vi "MB_TCP_7024i.vi"(5 "Status Reference":T1, 6 "N":i32, 7 "Data Reference":T2, 9 "timeouts":T3={"conn_timeout"=1000, "reconn_timeout"=3000, "N attempt max"=3, "t_reset_TTL"=120000, "write_timeout"=10, "read_timeout"=500, "period"=100} {"t_reset_TTL" min=10 max=240000 step=1; "period" min=10 max=100000 step=1; "read_timeout" min=10 max=60000 step=1; "write_timeout" min=1 max=60000 step=1; "N attempt max" min=1 max=5 step=1; "reconn_timeout" min=10 max=240000 step=1; "conn_timeout" min=10 max=240000}, 10 "write enable":bool=TRUE, 11 "stop":bool) -> (0 "error out":errorcluster, 2 "errors":i32, 3 "Z3":u32)   [LabVIEW 2019, in "MB_TCP1.lvlib"]
uses:
  MB_TCP1.lvlib
  Timer Delay/Timers.lvlib
  NI_modbus_upd/NI_modbus_upd.lvlib
  NI_modbus_upd/MB Modbus Command.ctl
  ICPCON Registers/ICPCON Registers.lvlib
  ICPCON Status/ICPCON Status.lvlib
  Timer Delay/unix time 1ms.vi
  NI_modbus_upd/TCP/TCP.lvclass
  ICPCON Status/Ctl/ICPCON Status.ctl
  ICPCON Registers/Ctl/ICPCON Data.ctl
panel:
  out "stopped":bool
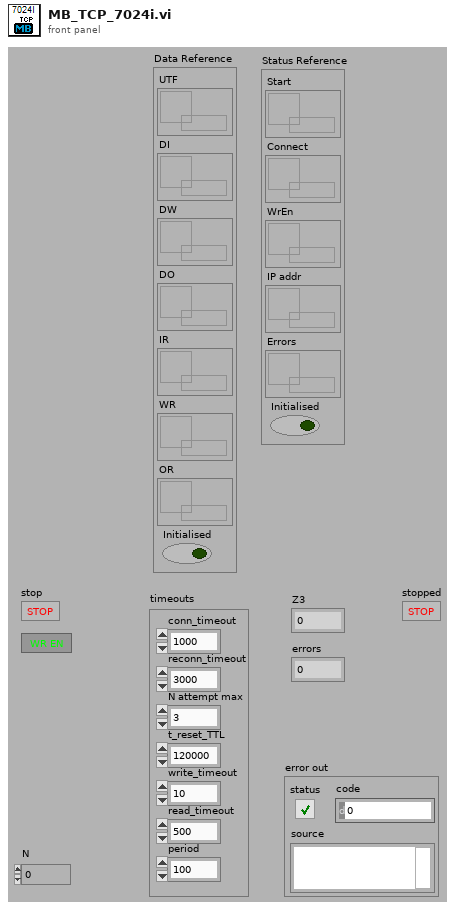
[diagram p1: front panel]
types:
  T1 = typedef "ICPCON Status.lvlib/ICPCON Status.ctl" = cluster{"Start":refnum<data-value>, "Connect":refnum<data-value>, "WrEn":refnum<data-value>, "IP addr":refnum<data-value>, "Errors":refnum<data-value>, "Initialised":bool}
  T2 = typedef "ICPCON Registers.lvlib/ICPCON Data.ctl" = cluster{"UTF":refnum<data-value>, "DI":refnum<data-value>, "DW":refnum<data-value>, "DO":refnum<data-value>, "IR":refnum<data-value>, "WR":refnum<data-value>, "OR":refnum<data-value>, "Initialised":bool}
  T3 = cluster{"conn_timeout":i32, "reconn_timeout":i32, "N attempt max":i32, "t_reset_TTL":i32, "write_timeout":i32, "read_timeout":i32, "period":i32}
  T4 = cluster{"Transaction ID":u16, "Protocol ID":u16, "Length":u16, "Unit ID":u8}
  T5 = typedef "NI_modbus_upd.lvlib/MB Modbus Command.ctl" = cluster{"Function Code":u8, "Starting Address":u16, "Quantity":u16, "Data":u16[], "Discrete":bool[]}
  T6 = cluster{"Remote IP Address":string, "Remote Port":u16}
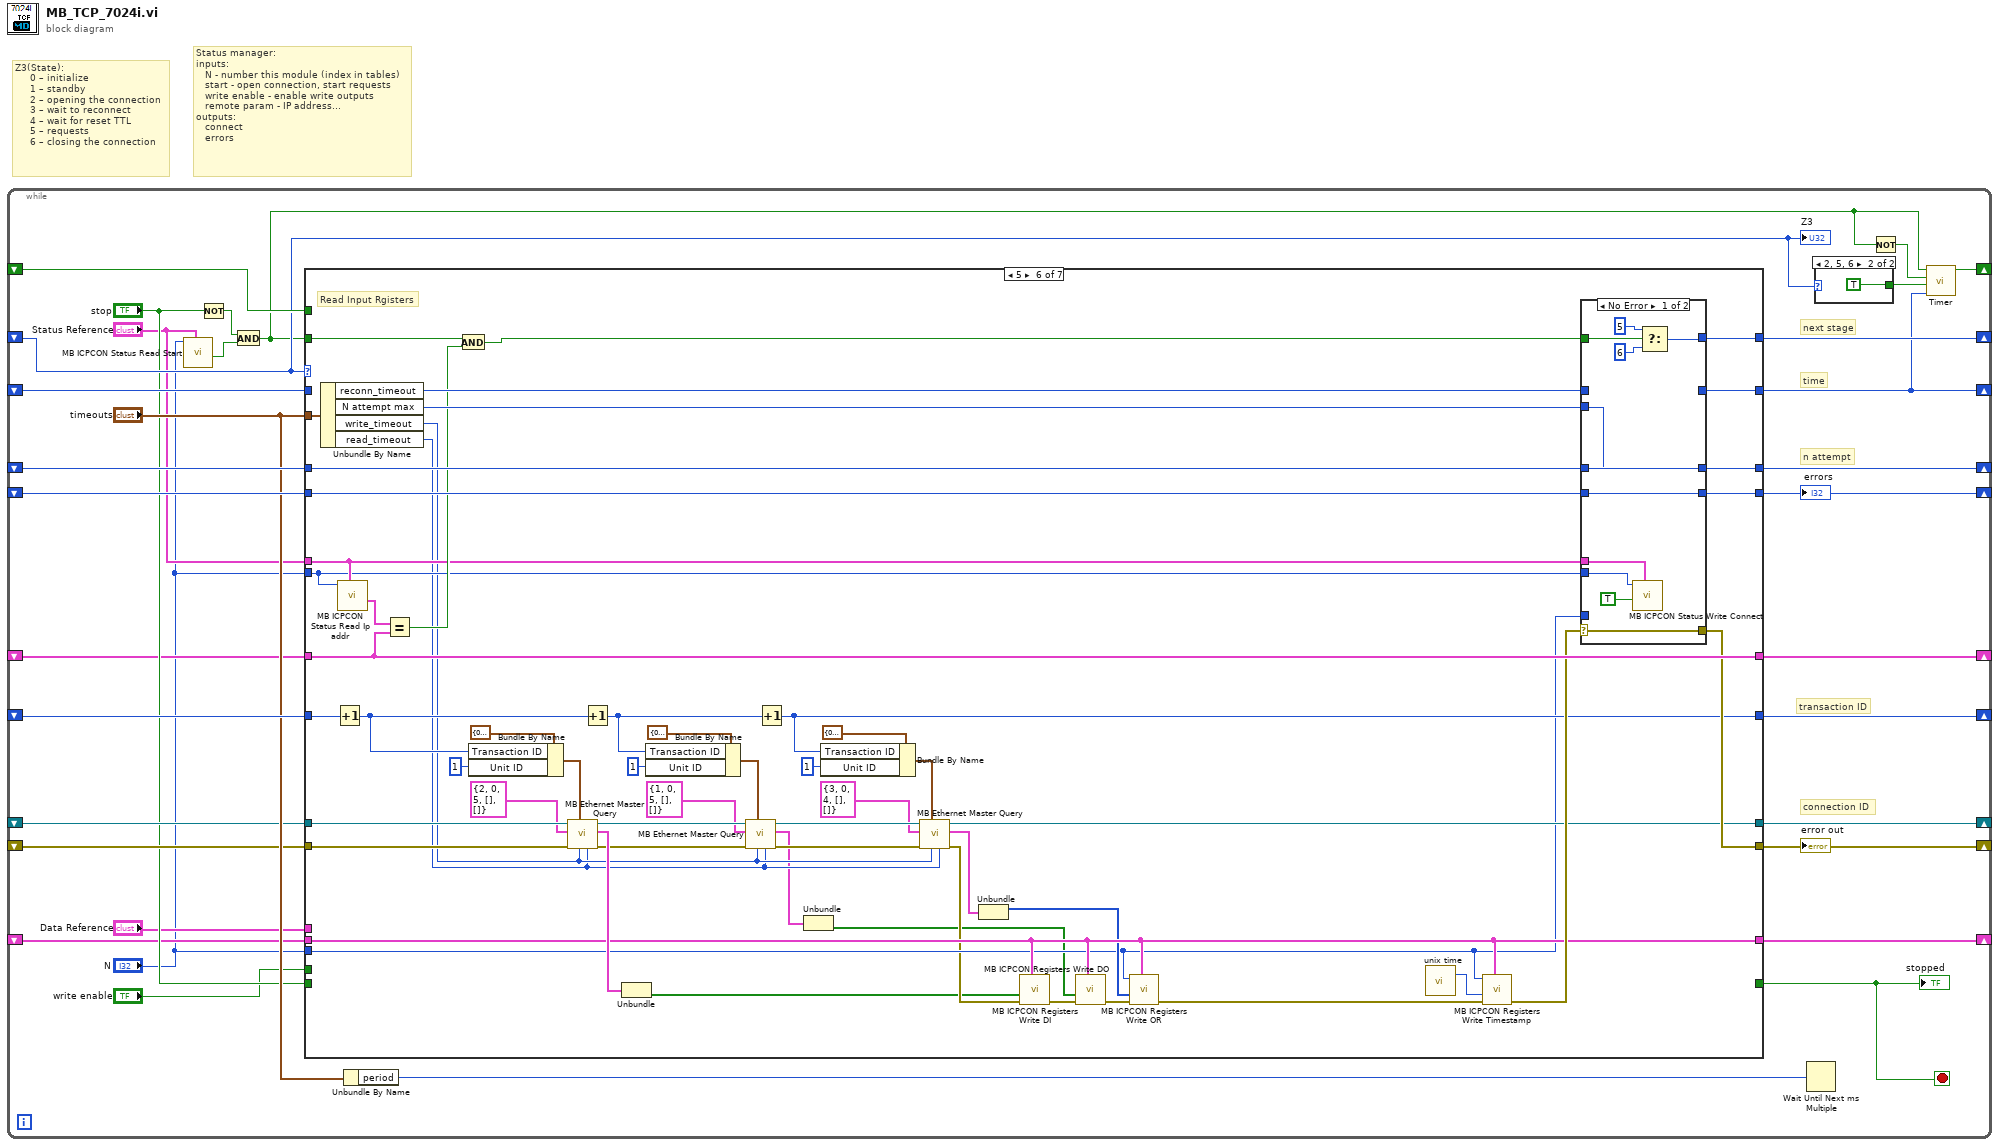
[diagram p0: block diagram]
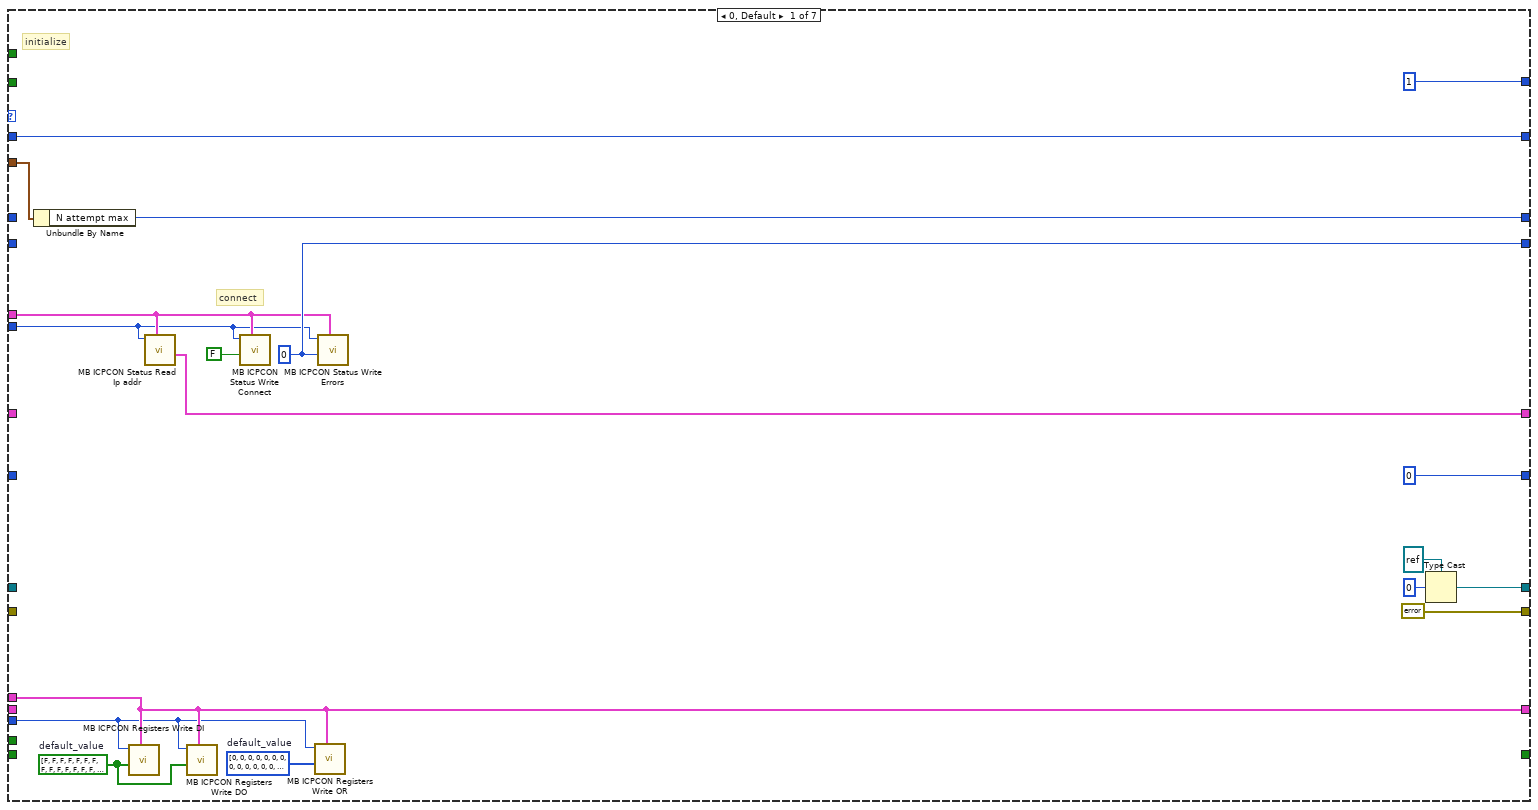
[diagram p2: hidden frame]
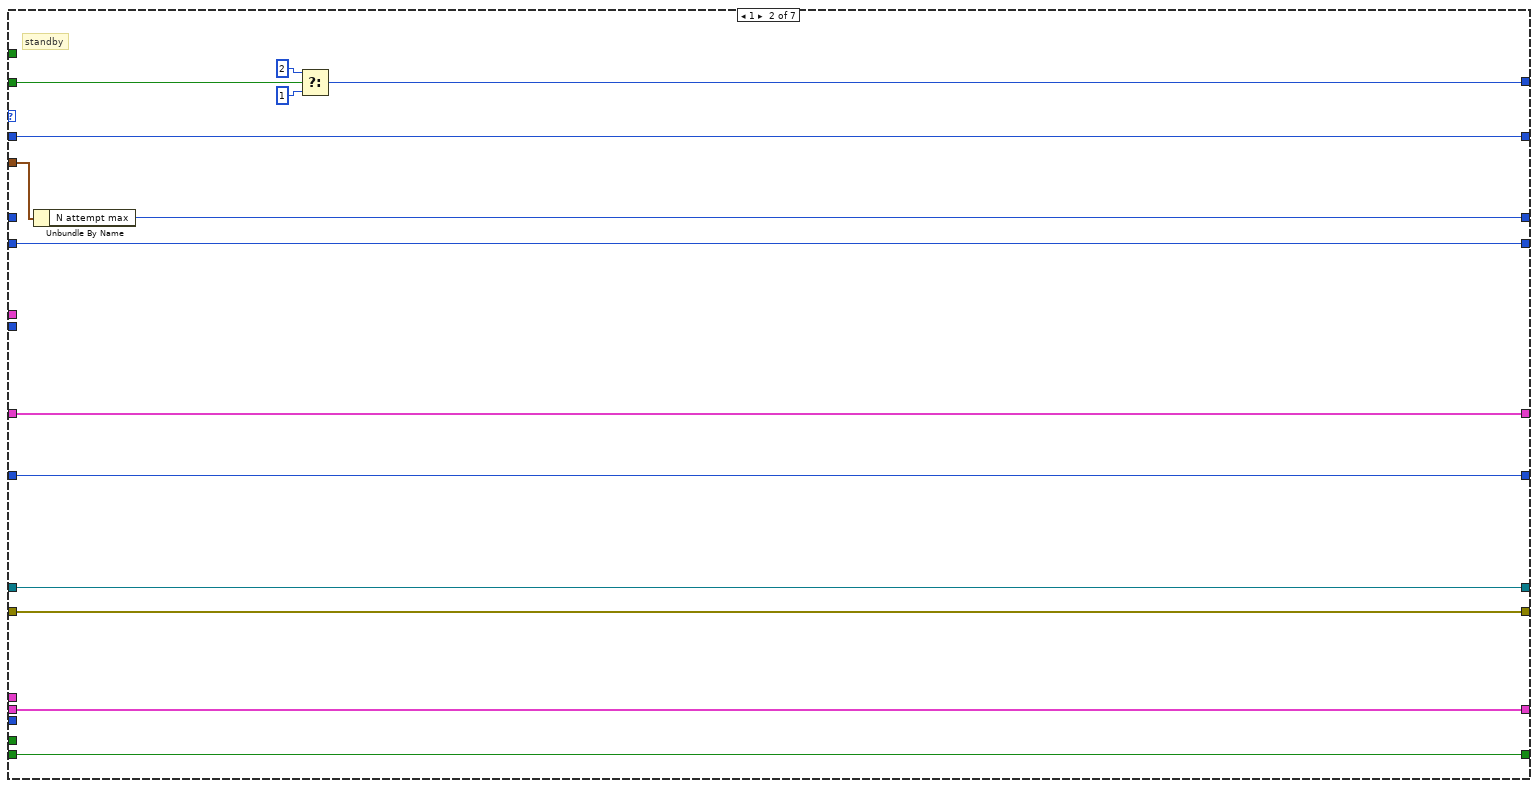
[diagram p3: hidden frame]
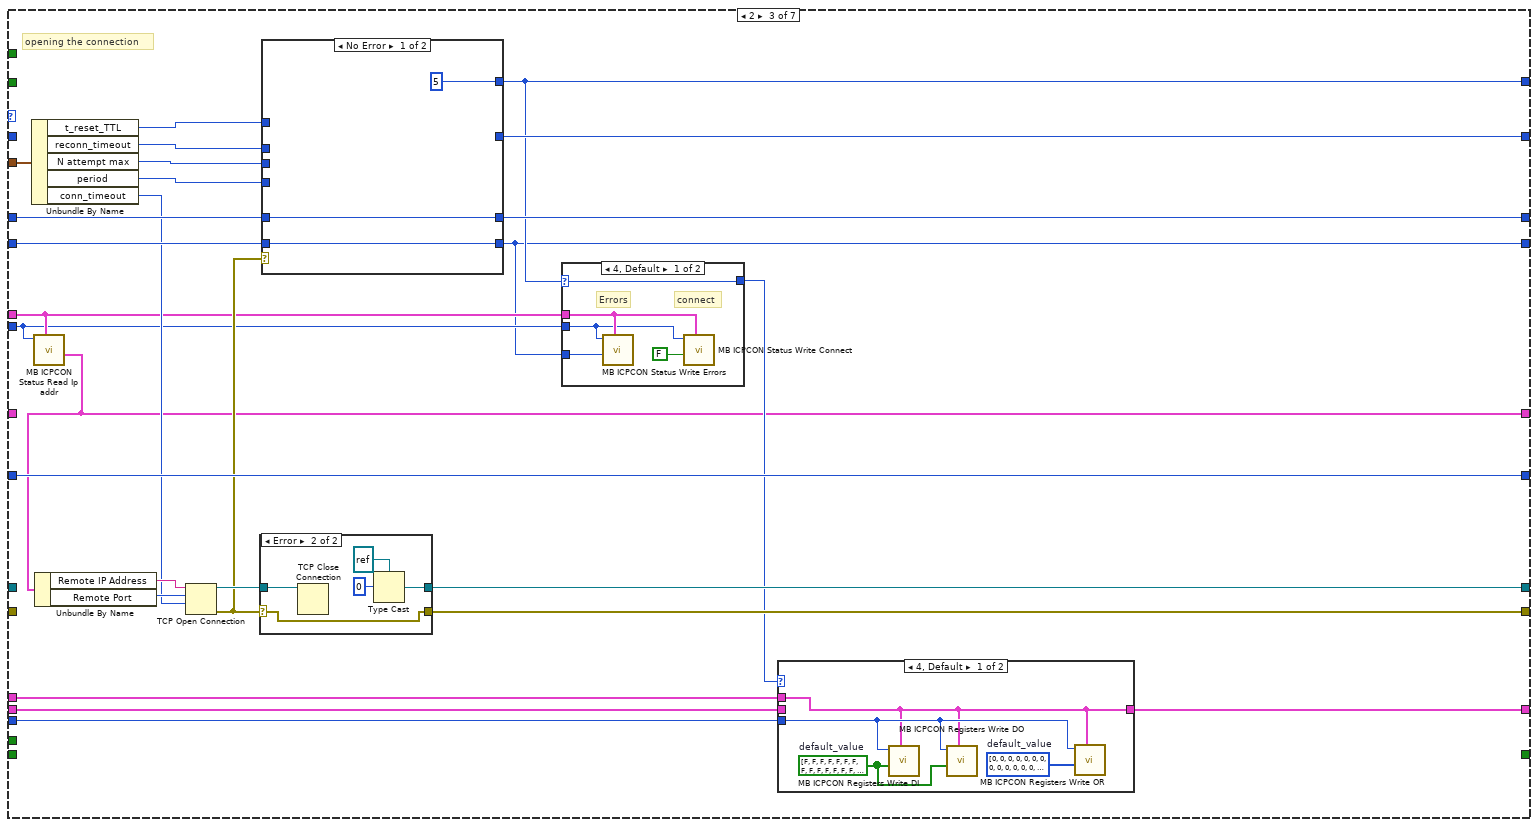
[diagram p4: hidden frame]
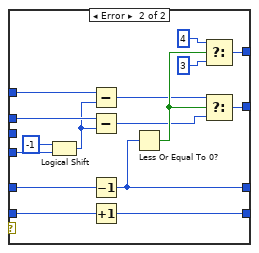
[diagram p8: hidden frame]
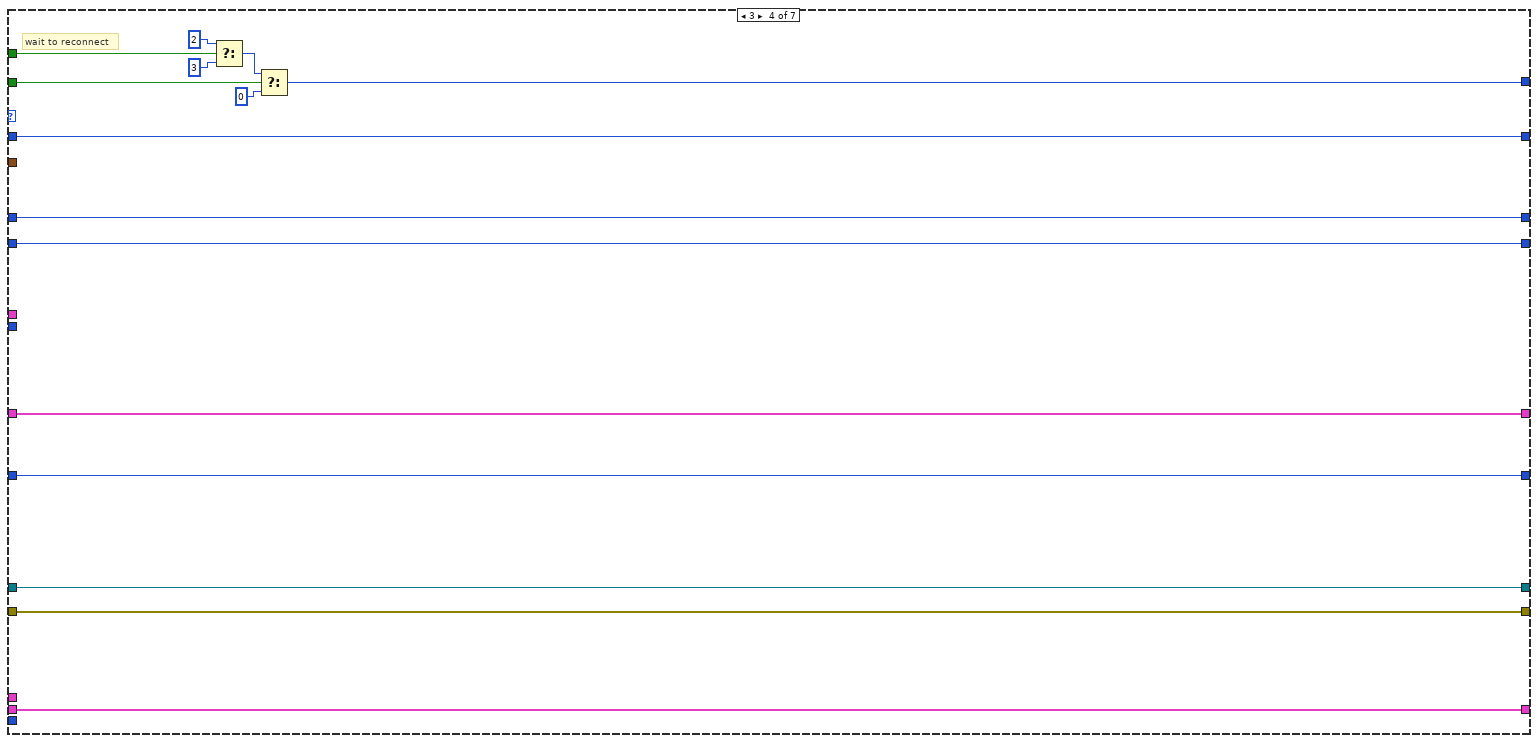
[diagram p9: hidden frame]
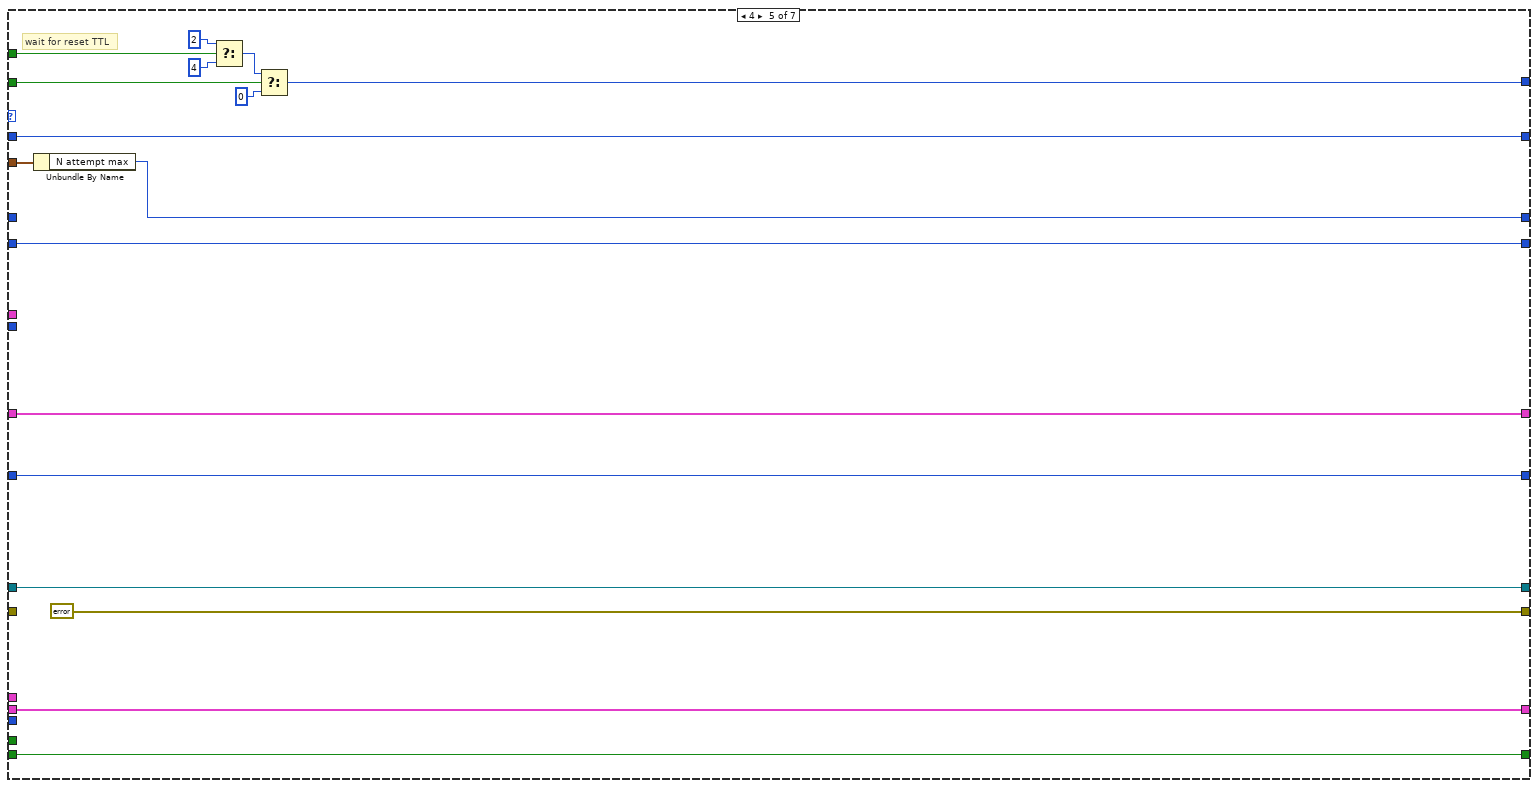
[diagram p10: hidden frame]
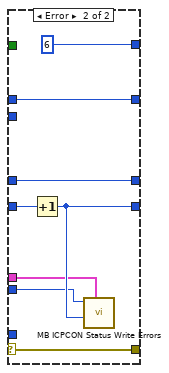
[diagram p11: hidden frame]
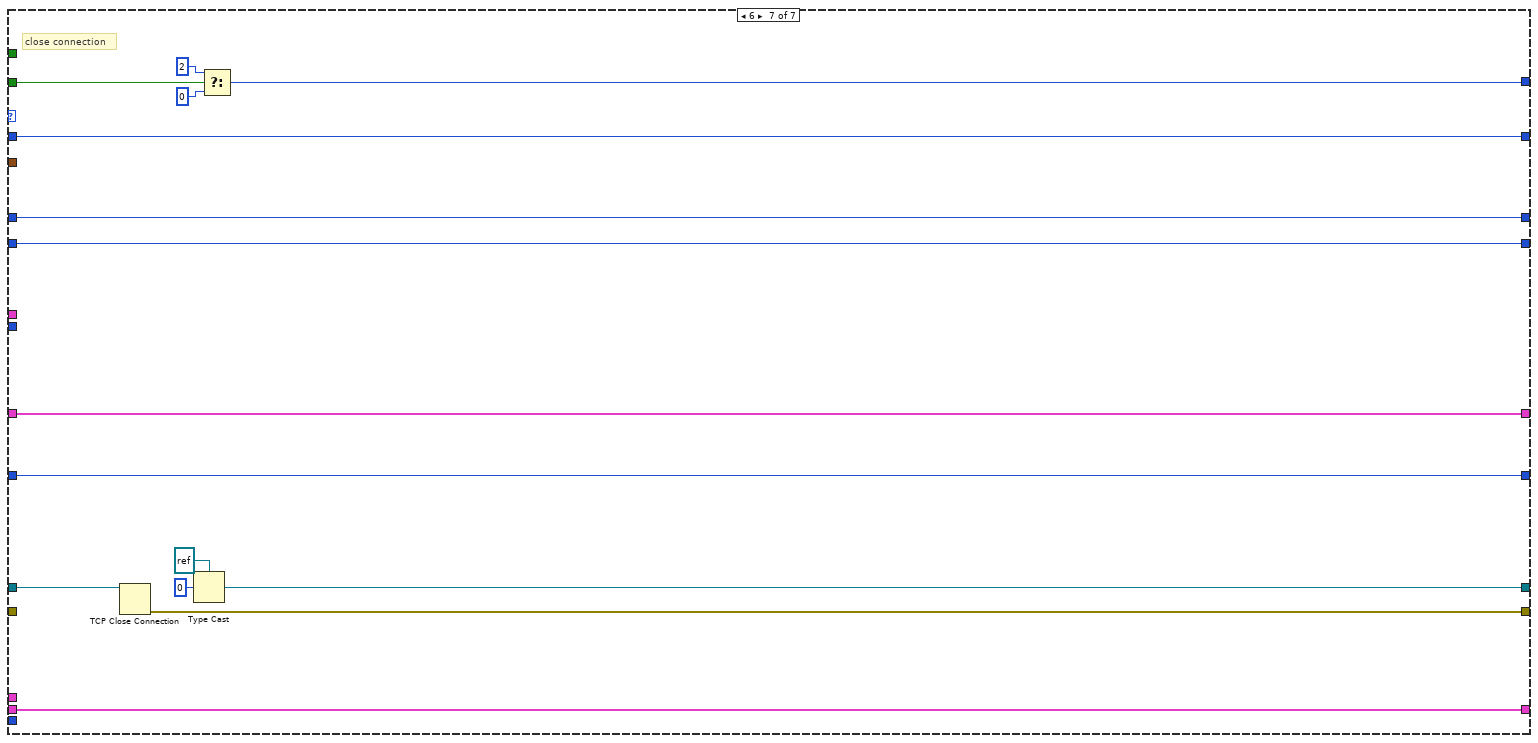
[diagram p12: hidden frame]
diagram:
  # "Status manager:\ninputs:\n   N - number this module (index in tables)\n   start - open connection, start requests\n   write enable - enable write outputs\n   remote param - IP address...\noutputs:\n   connect\n   errors"
  # "Z3(State):\n     0 – initialize \n     1 – standby\n     2 – opening the connection\n     3 – wait to reconnect\n     4 – wait for reset TTL\n     5 – requests\n     6 – closing the connection"
  n1 = while {
    shift-right: [w18] -> _
    shift-left: _ -> [w14]
    shift-right: [w17] -> _
    shift-left: _ -> [w32]
    shift-right: [w31] -> _
    shift-left: _ -> [w29]
    shift-right: [w30] -> _
    shift-left: _ -> [w28]
    shift-right: [w27] -> _
    shift-left: _ -> [w19]
    shift-right: [w26] -> _
    shift-left: _ -> [w20]
    shift-right: [w25] -> _
    shift-left: _ -> [w24]
    shift-right: [w16] -> _
    shift-left: _ -> [w15]
    shift-right: [w10] -> _
    shift-left: _ -> [w9]
    shift-right: [w7] -> _
    shift-left: _ -> [w6]
    stop <- w1 stop-if-true
    # "connection ID"
    # "transaction ID"
    # "n attempt"
    # "time"
    # "next stage"
    n2 = call "MB ICPCON Status Read Start.vi"("Status Reference"="Status Reference", "N"="N") -> ("Start"=w4:bool)  [unwired: 8 in, 1 out]
    n3 = Not(x="stop") -> (.not. x?=w12:bool)
    n4 = And(x=w12, y=w4) -> (x .and. y?=w13:bool)
    n5 = case shown="5" w14 {
      tunnel: [w49 w57 w78 w142 w147 w177 w247] -> w27
      tunnel: [errorcluster {"status"=FALSE, "code"=0, "source"=""} ("error out") w56 w76 w141 errorcluster {"status"=FALSE, "code"=0, "source"=""} ("error out") w191 w248] -> w26
      tunnel: w19 -> [_ w57 _ w142 w147 w207 w244]
      tunnel: w20 -> [_ w56 _ w141 _ w206 _]
      tunnel: w24 -> [_ w65 w92 w144 w161 w216 w249]
      tunnel: [u16 0 ("x") w65 w92 w144 w161 w174 w249] -> w25
      tunnel: [w44 w61 w88 w143 w157 w214 w241] -> w31
      tunnel: w29 -> [_ _ w89 w143 _ w214 w241]
      tunnel: [w39 w64 w66 w140 w160 w213 w246] -> w30
      tunnel: w28 -> [_ w64 w91 w140 w160 w212 w246]
      tunnel: [w46 w63 w85 w139 w159 w209 w245] -> w17
      tunnel: w32 -> [w46 w63 _ w139 w159 _ w245]
      tunnel: "timeouts" -> [w45 w62 w90 _ w158 w215 _]
      tunnel: w13 -> [_ w55 _ w135 w149 w201 w242]
      tunnel: [u32 1 w58 w75 w132 w152 w208 w237] -> w18
      tunnel: w15 -> [_ _ _ w133 w151 _ _]
      tunnel: "N" -> [w35 _ w72 _ _ w168 _]
      tunnel: "stop" -> [_ w54 _ _ w148 _ _]
      tunnel: [_ w54 _ _ w148 _ _] -> w1
      tunnel: [w40 w53 w69 w131 w146 w199 w236] -> w10
      tunnel: w9 -> [_ w53 _ w131 w146 w199 w236]
      tunnel: "Data Reference" -> [w36 _ w71 _ _ _ _]
      tunnel: [w36 w52 w74 w130 w145 w171 w235] -> w7
      tunnel: w6 -> [_ w52 w70 w130 w145 w171 w235]
      tunnel: "write enable" -> [_ _ _ _ _ _ _]
      tunnel: "Status Reference" -> [w38 _ w68 _ _ w187 _]
      tunnel: "N" -> [w37 _ w67 _ _ w186 _]
      frame 0, Default {
        w39 = 0 ("N attempt max")
        w34 = bool[] [FALSE, FALSE, FALSE, FALSE, FALSE, FALSE, FALSE, FALSE, FALSE, FALSE, FALSE, FALSE, FALSE, FALSE, FALSE, FALSE, FALSE, FALSE, FALSE, FALSE, FALSE, FALSE, FALSE, FALSE, FALSE, FALSE, FALSE, FALSE, FALSE, FALSE, FALSE, FALSE]  # default_value
        w42 = u16[] [0, 0, 0, 0, 0, 0, 0, 0, 0, 0, 0, 0, 0, 0, 0, 0, 0, 0, 0, 0]  # default_value
        # "connect"
        # "initialize"
        n6 = Unbundle By Name(w45) -> ("N attempt max"=w44:i32)
        n7 = call "MB ICPCON Registers Write DI.vi"("Data Reference"=w36, "Bits In"=w34, "N"=w35) -> ()  [unwired: 8 in, 1 out]
        n8 = call "MB ICPCON Status Read Ip addr.vi"("Status Reference"=w38, "N"=w37) -> ("IP address"=w40:T6)  [unwired: 8 in, 1 out]
        n9 = call "MB ICPCON Registers Write DO.vi"("Data Reference"=w36, "Bits In"=w34, "N"=w35) -> ()  [unwired: 8 in, 1 out]
        n10 = call "MB ICPCON Status Write Connect.vi"("Status Reference"=w38, "Connect"=FALSE ("connect"), "N"=w37) -> ()  [unwired: 8 in, 1 out]
        n11 = call "MB ICPCON Registers Write OR.vi"("Data Reference"=w36, "Words In"=w42, "N"=w35) -> ()  [unwired: 8 in, 1 out]
        n12 = call "MB ICPCON Status Write Errors.vi"("Status Reference"=w38, "Errors"=w39, "N"=w37) -> ()  [unwired: 8 in, 1 out]
        n13 = Type Cast(type=refnum<k5> refnum ("connection ID"), x=u32 0) -> (*(type *) &x=w49:refnum<k5>)
      }
      frame 1 {
        # "standby"
        n14 = Unbundle By Name(w62) -> ("N attempt max"=w61:i32)
        n15 = Select(t=u32 2, s=w55, f=u32 1) -> (s? t:f=w58:u32)
      }
      frame 2 {
        # "opening the connection"
        n16 = Unbundle By Name(w90) -> ("t_reset_TTL"=w84:i32, "reconn_timeout"=w86:i32, "N attempt max"=w87:i32, "period"=w81:i32, "conn_timeout"=w80:i32)
        n17 = call "MB ICPCON Status Read Ip addr.vi"("Status Reference"=w68, "N"=w67) -> ("IP address"=w69:T6)  [unwired: 8 in, 1 out]
        n18 = Unbundle By Name(w69) -> ("Remote IP Address"=w83:string, "Remote Port"=w82:u16)
        n19 = TCP Open Connection(address=w83, remote port or service name=w82, timeout ms (60000)=w80) -> (connection ID=w79:refnum<k5>, error out=w77:errorcluster)  [unwired: 2 in]
        n20 = case shown="Error" w77 {
          selector: w77 -> [w104 w106]
          tunnel: w79 -> [w105 w109]
          tunnel: [w105 w108] -> w78
          tunnel: [w104 w106] -> w76
          frame No Error {
          }
          frame Error {
            n21 = TCP Close Connection(connection ID=w109) -> ()  [unwired: 2 in, 2 out]
            n22 = Type Cast(type=refnum<k5> refnum ("connection ID"), x=u32 0) -> (*(type *) &x=w108:refnum<k5>)
          }
        }
        n23 = case shown="No Error" w77 {
          tunnel: w91 -> [w113 w129]
          tunnel: [w113 w128] -> w66
          tunnel: w89 -> [w112 w127]
          tunnel: [w112 w126] -> w88
          tunnel: w87 -> [_ _]
          tunnel: [u32 5 w123] -> w75
          tunnel: w86 -> [_ w122]
          tunnel: [_ w121] -> w85
          tunnel: w84 -> [_ w118]
          tunnel: w81 -> [_ w116]
          frame No Error {
          }
          frame Error {
            n24 = Logical Shift(y=i16 -1, x=w116) -> (x << y=w114:i32)
            n25 = Subtract(x=w118, y=w114) -> (x-y=w117:i32)
            n26 = Subtract(x=w122, y=w114) -> (x-y=w119:i32)
            n27 = Decrement(x=w127) -> (x-1=w126:i32)
            n28 = Increment(x=w129) -> (x+1=w128:i32)
            n29 = Less Or Equal To 0?(x=w126) -> (x <= 0?=w120:bool)
            n30 = Select(t=u32 4, s=w120, f=u32 3) -> (s? t:f=w123:u32)
            n31 = Select(t=w117, s=w120, f=w119) -> (s? t:f=w121:i32)
          }
        }
        n32 = case shown="4, Default" w75 {
          selector: w75 -> [w102 w103]
          tunnel: [w102 w103] -> w73
          tunnel: w68 -> [w100 _]
          tunnel: w67 -> [w99 _]
          tunnel: w66 -> [w98 _]
          frame 4, Default {
            # "Errors"
            # "connect"
            n33 = call "MB ICPCON Status Write Errors.vi"("Status Reference"=w100, "Errors"=w98, "N"=w99) -> ()  [unwired: 8 in, 1 out]
            n34 = call "MB ICPCON Status Write Connect.vi"("Status Reference"=w100, "Connect"=FALSE ("f"), "N"=w99) -> ()  [unwired: 8 in, 1 out]
          }
          frame 3, 5 {
          }
        }
        n35 = case shown="4, Default" w73 {
          tunnel: w72 -> [w94 _]
          tunnel: w70 -> [_ w97]
          tunnel: [w93 w97] -> w74
          tunnel: w71 -> [w93 _]
          frame 4, Default {
            w95 = bool[] [FALSE, FALSE, FALSE, FALSE, FALSE, FALSE, FALSE, FALSE, FALSE, FALSE, FALSE, FALSE, FALSE, FALSE, FALSE, FALSE, FALSE, FALSE, FALSE, FALSE, FALSE, FALSE, FALSE, FALSE, FALSE, FALSE, FALSE, FALSE, FALSE, FALSE, FALSE, FALSE]  # default_value
            w96 = u16[] [0, 0, 0, 0, 0, 0, 0, 0, 0, 0, 0, 0, 0, 0, 0, 0, 0, 0, 0, 0]  # default_value
            n36 = call "MB ICPCON Registers Write DI.vi"("Data Reference"=w93, "Bits In"=w95, "N"=w94) -> ()  [unwired: 8 in, 1 out]
            n37 = call "MB ICPCON Registers Write DO.vi"("Data Reference"=w93, "Bits In"=w95, "N"=w94) -> ()  [unwired: 8 in, 1 out]
            n38 = call "MB ICPCON Registers Write OR.vi"("Data Reference"=w93, "Words In"=w96, "N"=w94) -> ()  [unwired: 8 in, 1 out]
          }
          frame 3, 5 {
          }
        }
      }
      frame 3 {
        # "wait to reconnect"
        n39 = Select(t=u32 2, s=w133, f=u32 3) -> (s? t:f=w134:u32)
        n40 = Select(t=w134, s=w135, f=u32 0) -> (s? t:f=w132:u32)
      }
      frame 4 {
        # "wait for reset TTL"
        n41 = Unbundle By Name(w158) -> ("N attempt max"=w157:i32)
        n42 = Select(t=u32 2, s=w151, f=u32 4) -> (s? t:f=w153:u32)
        n43 = Select(t=w153, s=w149, f=u32 0) -> (s? t:f=w152:u32)
      }
      frame 5 {
        # "Read Input Rgisters"
        n44 = Unbundle By Name(w215) -> ("reconn_timeout"=w210:i32, "N attempt max"=w211:i32, "write_timeout"=w180:i32, "read_timeout"=w179:i32)
        n45 = Increment(x=w216) -> (x+1=w194:u16)
        n46 = call "MB ICPCON Status Read Ip addr.vi"("Status Reference"=w187, "N"=w186) -> ("IP address"=w188:T6)  [unwired: 8 in, 1 out]
        n47 = Equal?(x=w188, y=w199) -> (x = y?=w198:bool)
        n48 = And(x=w201, y=w198) -> (x .and. y?=w200:bool)
        n49 = Bundle By Name(cluster=T4 {"Transaction ID"=0, "Protocol ID"=0, "Length"=0, "Unit ID"=0} ("MBAP Header"), "Transaction ID"=w194, "Unit ID"=u8 1) -> (w202:T4)
        n50 = call "MB Ethernet Master Query.vi"(4:w179, 6:w180, "MBAP Header"=w202, "error in (no error)"=w206, "Modbus Command"=T5 {"Function Code"=2, "Starting Address"=0, "Quantity"=5, "Data"=[], "Discrete"=[]}, "TCP in"=w207) -> ("error out"=w193:errorcluster, "Registers"=w205:cluster{"Registers":u16[], "Discrete":bool[]}, "TCP out"=w192:refnum<class "TCP.lvclass">)  [unwired: 2 in, 1 out]
        n51 = Increment(x=w194) -> (x+1=w175:u16)
        n52 = Unbundle(w205) -> ("Discrete"=w162:bool[])  [unwired: 1 out]
        n53 = Bundle By Name(cluster=T4 {"Transaction ID"=0, "Protocol ID"=0, "Length"=0, "Unit ID"=0} ("MBAP Header"), "Transaction ID"=w175, "Unit ID"=u8 1) -> (w197:T4)
        n54 = call "MB Ethernet Master Query.vi"(4:w179, 6:w180, "MBAP Header"=w197, "error in (no error)"=w193, "Modbus Command"=T5 {"Function Code"=1, "Starting Address"=0, "Quantity"=5, "Data"=[], "Discrete"=[]} ("MODBUS Command"), "TCP in"=w192) -> ("error out"=w176:errorcluster, "Registers"=w172:cluster{"Registers":u16[], "Discrete":bool[]}, "TCP out"=w178:refnum<class "TCP.lvclass">)  [unwired: 2 in, 1 out]
        n55 = Increment(x=w175) -> (x+1=w174:u16)
        n56 = Unbundle(w172) -> ("Discrete"=w163:bool[])  [unwired: 1 out]
        n57 = Bundle By Name(cluster=T4 {"Transaction ID"=0, "Protocol ID"=0, "Length"=0, "Unit ID"=0} ("MBAP Header"), "Transaction ID"=w174, "Unit ID"=u8 1) -> (w181:T4)
        n58 = call "MB Ethernet Master Query.vi"(4:w179, 6:w180, "MBAP Header"=w181, "error in (no error)"=w176, "Modbus Command"=T5 {"Function Code"=3, "Starting Address"=0, "Quantity"=4, "Data"=[], "Discrete"=[]} ("MODBUS Command"), "TCP in"=w178) -> ("error out"=w167:errorcluster, "Registers"=w170:cluster{"Registers":u16[], "Discrete":bool[]}, "TCP out"=w177:refnum<class "TCP.lvclass">)  [unwired: 2 in, 1 out]
        n59 = Unbundle(w170) -> ("Registers"=w169:u16[])  [unwired: 1 out]
        n60 = call "MB ICPCON Registers Write DI.vi"("Data Reference"=w171, "error in (no error)"=w167, "Bits In"=w162) -> ("error out"=w166:errorcluster)  [unwired: 8 in]
        n61 = call "MB ICPCON Registers Write DO.vi"("Data Reference"=w171, "error in (no error)"=w166, "Bits In"=w163) -> ("error out"=w165:errorcluster)  [unwired: 8 in]
        n62 = call "MB ICPCON Registers Write OR.vi"("Data Reference"=w171, "error in (no error)"=w165, "Words In"=w169, "N"=w168) -> ("error out"=w164:errorcluster)  [unwired: 7 in]
        n63 = call-poly "unix time.vi"() -> ("unix time (ms)"=w189:u64)  [unwired: 2 in, 1 out]
        n64 = call "MB ICPCON Registers Write Timestamp.vi"("Data Reference"=w171, "error in (no error)"=w164, "UTF"=w189, "N"=w168) -> ("error out"=w190:errorcluster)  [unwired: 7 in]
        n65 = case shown="No Error" w190 {
          selector: w190 -> [w220 w230]
          tunnel: w212 -> [w221 w234]
          tunnel: [w221 w229] -> w213
          tunnel: [w223 u32 6] -> w208
          tunnel: w214 -> [_ w232]
          tunnel: w211 -> [w226 _]
          tunnel: [w226 w232] -> _
          tunnel: w210 -> [_ w231]
          tunnel: [_ w231] -> w209
          tunnel: w200 -> [w222 _]
          tunnel: w168 -> [_ _]
          tunnel: [w220 w230] -> w191
          tunnel: w187 -> [w218 w228]
          tunnel: w186 -> [w217 w227]
          frame No Error {
            n66 = call "MB ICPCON Status Write Connect.vi"("Status Reference"=w218, "Connect"=TRUE ("f"), "N"=w217) -> ()  [unwired: 8 in, 1 out]
            n67 = Select(t=u32 5, s=w222, f=u32 6) -> (s? t:f=w223:u32)
          }
          frame Error {
            n68 = Increment(x=w234) -> (x+1=w229:i32)
            n69 = call "MB ICPCON Status Write Errors.vi"("Status Reference"=w228, "Errors"=w229, "N"=w227) -> ()  [unwired: 8 in, 1 out]
          }
        }
      }
      frame 6 {
        # "close connection"
        n70 = TCP Close Connection(connection ID=w244) -> (error out=w248:errorcluster)  [unwired: 2 in, 1 out]
        n71 = Type Cast(type=refnum<k5> refnum ("connection ID"), x=u32 0) -> (*(type *) &x=w247:refnum<k5>)
        n72 = Select(t=u32 2, s=w242, f=u32 0) -> (s? t:f=w237:u32)
      }
    }
    "error out" <- w26
    "errors" <- w30
    "stopped" <- w1
    n73 = Unbundle By Name("timeouts") -> ("period"=w22:i32)
    n74 = Wait Until Next ms Multiple(millisecond multiple=w22) -> ()  [unwired: 1 out]
    n75 = case shown="2, 5, 6" w14 {
      tunnel: [_ TRUE] -> w21
      frame 0, Default {
      }
      frame 2, 5, 6 {
      }
    }
    n76 = Not(x=w13) -> (.not. x?=w33:bool)
    n77 = call "Timer.vi"("ms"=w17, "Load (F)"=w21, "Reset (F)"=w33, "Start (T)"=w13) -> ("End"=w16:bool)  [unwired: 5 in, 1 out]
    "Z3" <- w14
  }
